vi "Format Pin Name In Error Message.vi"(0 "Pin Name":string[](array[string]), 2 "Parameter Name":string, 5 "Error[]":bool[](array[boolean]), 11 "error in":errorcluster) -> (4 "Error Message":string, 15 "error out":errorcluster)   [LabVIEW 2024, in "devicePowerSequencerCoreLogic.lvlib"]
uses:
  devicePowerSequencerCoreLogic.lvlib
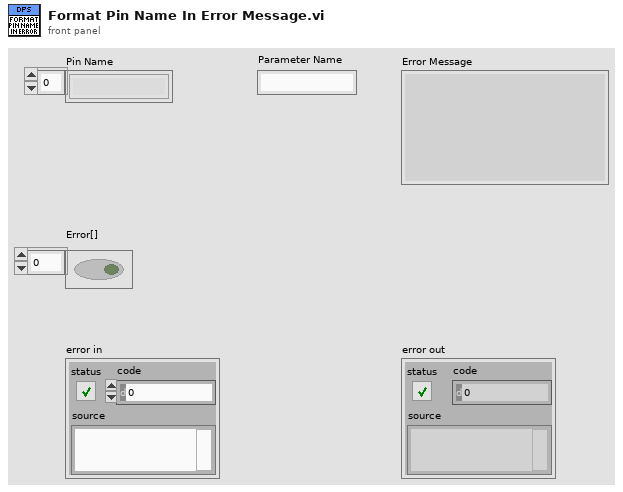
[diagram p1: front panel]
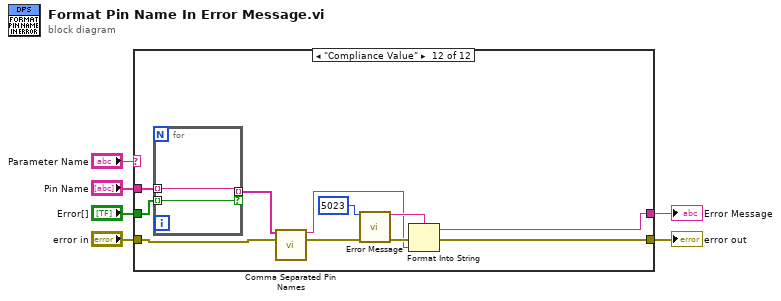
[diagram p0: block diagram]
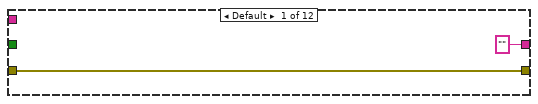
[diagram p2: hidden frame]
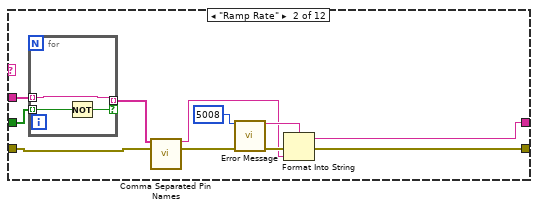
[diagram p3: hidden frame]
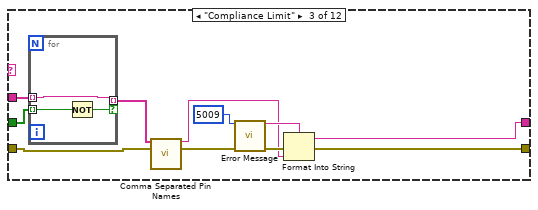
[diagram p4: hidden frame]
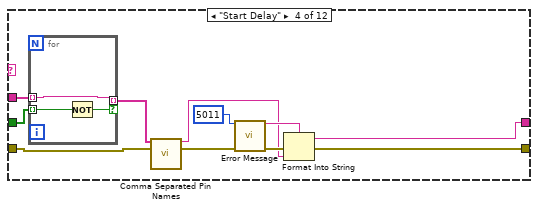
[diagram p5: hidden frame]
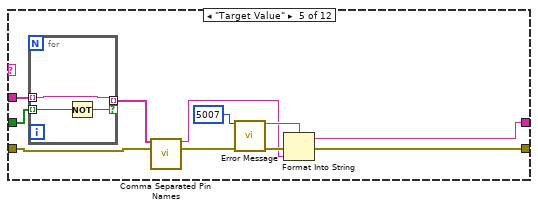
[diagram p6: hidden frame]
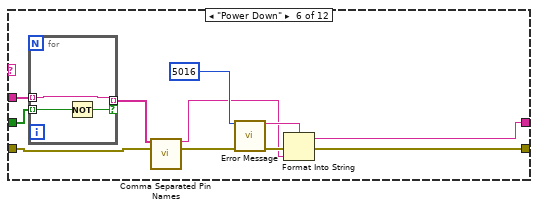
[diagram p7: hidden frame]
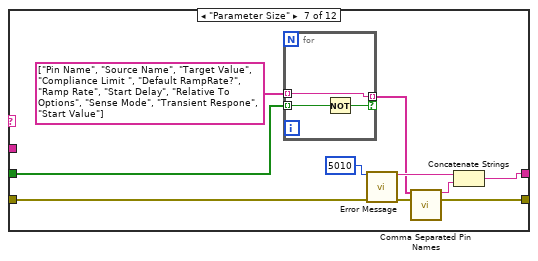
[diagram p8: hidden frame]
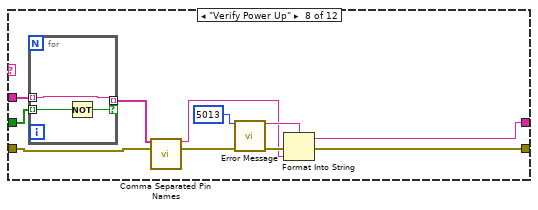
[diagram p9: hidden frame]
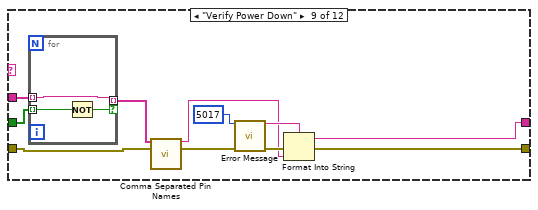
[diagram p10: hidden frame]
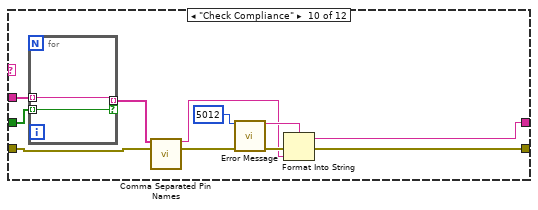
[diagram p11: hidden frame]
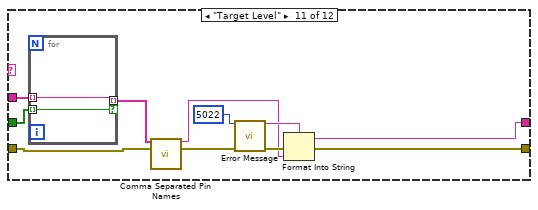
[diagram p12: hidden frame]
diagram:
  n1 = case shown="\"Compliance Value\"" "Parameter Name" {
    tunnel: "Pin Name" -> [_ w19 w33 w47 w61 w75 _ w102 w116 w130 w143 w156]
    tunnel: "Error[]" -> [_ w18 w32 w46 w60 w74 w86 w101 w115 w129 w142 w155]
    tunnel: ["" w17 w31 w45 w59 w73 w87 w100 w114 w128 w141 w154] -> w3
    tunnel: [w7 w16 w30 w44 w58 w72 w80 w99 w113 w127 w140 w153] -> w2
    tunnel: "error in" -> [w7 w9 w23 w37 w51 w65 w83 w92 w108 w120 w133 w146]
    frame Default {
    }
    frame "Ramp Rate" {
      n2 = for {
        tunnel: w19 -> [w22] mode=indexing
        tunnel: w18 -> [w21] mode=indexing
        tunnel: [w22] -> w12 mode=indexing if=w20
        n3 = Not(x=w21) -> (.not. x?=w20:bool)
      }
      n4 = call "Comma Separated Pin Names.vi"("Pin Names"=w12, "error in (no error)"=w9) -> ("PinNames OUT"=w11:string, "error out"=w10:errorcluster)  [unwired: 12 in]
      n5 = call "Error Message.vi"("Error Code"=5008, "error in (no error)"=w10) -> ("Error Message"=w13:string, "error out"=w14:errorcluster)  [unwired: 11 in, 1 out]
      n6 = Format Into String(format string=w13, error in=w14, w11) -> (resulting string=w17:string, error out=w16:errorcluster)  [unwired: 1 in]
    }
    frame "Compliance Limit" {
      n7 = for {
        tunnel: w33 -> [w36] mode=indexing
        tunnel: w32 -> [w35] mode=indexing
        tunnel: [w36] -> w26 mode=indexing if=w34
        n8 = Not(x=w35) -> (.not. x?=w34:bool)
      }
      n9 = call "Comma Separated Pin Names.vi"("Pin Names"=w26, "error in (no error)"=w23) -> ("PinNames OUT"=w25:string, "error out"=w24:errorcluster)  [unwired: 12 in]
      n10 = call "Error Message.vi"("Error Code"=5009, "error in (no error)"=w24) -> ("Error Message"=w28:string, "error out"=w29:errorcluster)  [unwired: 11 in, 1 out]
      n11 = Format Into String(format string=w28, error in=w29, w25) -> (resulting string=w31:string, error out=w30:errorcluster)  [unwired: 1 in]
    }
    frame "Start Delay" {
      n12 = for {
        tunnel: w47 -> [w50] mode=indexing
        tunnel: w46 -> [w49] mode=indexing
        tunnel: [w50] -> w40 mode=indexing if=w48
        n13 = Not(x=w49) -> (.not. x?=w48:bool)
      }
      n14 = call "Comma Separated Pin Names.vi"("Pin Names"=w40, "error in (no error)"=w37) -> ("PinNames OUT"=w39:string, "error out"=w38:errorcluster)  [unwired: 12 in]
      n15 = call "Error Message.vi"("Error Code"=5011, "error in (no error)"=w38) -> ("Error Message"=w41:string, "error out"=w42:errorcluster)  [unwired: 11 in, 1 out]
      n16 = Format Into String(format string=w41, error in=w42, w39) -> (resulting string=w45:string, error out=w44:errorcluster)  [unwired: 1 in]
    }
    frame "Target Value" {
      n17 = for {
        tunnel: w61 -> [w64] mode=indexing
        tunnel: w60 -> [w63] mode=indexing
        tunnel: [w64] -> w54 mode=indexing if=w62
        n18 = Not(x=w63) -> (.not. x?=w62:bool)
      }
      n19 = call "Comma Separated Pin Names.vi"("Pin Names"=w54, "error in (no error)"=w51) -> ("PinNames OUT"=w53:string, "error out"=w52:errorcluster)  [unwired: 12 in]
      n20 = call "Error Message.vi"("Error Code"=5007, "error in (no error)"=w52) -> ("Error Message"=w56:string, "error out"=w57:errorcluster)  [unwired: 11 in, 1 out]
      n21 = Format Into String(format string=w56, error in=w57, w53) -> (resulting string=w59:string, error out=w58:errorcluster)  [unwired: 1 in]
    }
    frame "Power Down" {
      n22 = for {
        tunnel: w75 -> [w78] mode=indexing
        tunnel: w74 -> [w77] mode=indexing
        tunnel: [w78] -> w68 mode=indexing if=w76
        n23 = Not(x=w77) -> (.not. x?=w76:bool)
      }
      n24 = call "Comma Separated Pin Names.vi"("Pin Names"=w68, "error in (no error)"=w65) -> ("PinNames OUT"=w67:string, "error out"=w66:errorcluster)  [unwired: 12 in]
      n25 = call "Error Message.vi"("Error Code"=5016, "error in (no error)"=w66) -> ("Error Message"=w70:string, "error out"=w71:errorcluster)  [unwired: 11 in, 1 out]
      n26 = Format Into String(format string=w70, error in=w71, w67) -> (resulting string=w73:string, error out=w72:errorcluster)  [unwired: 1 in]
    }
    frame "Parameter Size" {
      n27 = for {
        tunnel: w86 -> [w90] mode=indexing
        tunnel: string[] ["Pin Name", "Source Name", "Target Value", "Compliance Limit ", "Default RampRate?", "Ramp Rate", "Start Delay", "Relative To Options", "Sense Mode", "Transient Respone", "Start Value"] -> [w91] mode=indexing
        tunnel: [w91] -> w82 mode=indexing if=w89
        n28 = Not(x=w90) -> (.not. x?=w89:bool)
      }
      n29 = call "Error Message.vi"("Error Code"=5010, "error in (no error)"=w83) -> ("Error Message"=w84:string, "error out"=w79:errorcluster)  [unwired: 11 in, 1 out]
      n30 = call "Comma Separated Pin Names.vi"("Pin Names"=w82, "error in (no error)"=w79) -> ("PinNames OUT"=w81:string, "error out"=w80:errorcluster)  [unwired: 12 in]
      n31 = Concatenate Strings(w84, w81) -> (w87:string)
    }
    frame "Verify Power Up" {
      n32 = for {
        tunnel: w102 -> [w105] mode=indexing
        tunnel: w101 -> [w104] mode=indexing
        tunnel: [w105] -> w95 mode=indexing if=w103
        n33 = Not(x=w104) -> (.not. x?=w103:bool)
      }
      n34 = call "Comma Separated Pin Names.vi"("Pin Names"=w95, "error in (no error)"=w92) -> ("PinNames OUT"=w94:string, "error out"=w93:errorcluster)  [unwired: 12 in]
      n35 = call "Error Message.vi"("Error Code"=5013, "error in (no error)"=w93) -> ("Error Message"=w97:string, "error out"=w96:errorcluster)  [unwired: 11 in, 1 out]
      n36 = Format Into String(format string=w97, error in=w96, w94) -> (resulting string=w100:string, error out=w99:errorcluster)  [unwired: 1 in]
    }
    frame "Verify Power Down" {
      n37 = for {
        tunnel: w116 -> [w119] mode=indexing
        tunnel: w115 -> [w118] mode=indexing
        tunnel: [w119] -> w109 mode=indexing if=w117
        n38 = Not(x=w118) -> (.not. x?=w117:bool)
      }
      n39 = call "Comma Separated Pin Names.vi"("Pin Names"=w109, "error in (no error)"=w108) -> ("PinNames OUT"=w107:string, "error out"=w106:errorcluster)  [unwired: 12 in]
      n40 = call "Error Message.vi"("Error Code"=5017, "error in (no error)"=w106) -> ("Error Message"=w112:string, "error out"=w111:errorcluster)  [unwired: 11 in, 1 out]
      n41 = Format Into String(format string=w112, error in=w111, w107) -> (resulting string=w114:string, error out=w113:errorcluster)  [unwired: 1 in]
    }
    frame "Check Compliance" {
      n42 = for {
        tunnel: w130 -> [w132] mode=indexing
        tunnel: w129 -> [w131] mode=indexing
        tunnel: [w132] -> w123 mode=indexing if=w131
      }
      n43 = call "Comma Separated Pin Names.vi"("Pin Names"=w123, "error in (no error)"=w120) -> ("PinNames OUT"=w122:string, "error out"=w121:errorcluster)  [unwired: 12 in]
      n44 = call "Error Message.vi"("Error Code"=5012, "error in (no error)"=w121) -> ("Error Message"=w126:string, "error out"=w125:errorcluster)  [unwired: 11 in, 1 out]
      n45 = Format Into String(format string=w126, error in=w125, w122) -> (resulting string=w128:string, error out=w127:errorcluster)  [unwired: 1 in]
    }
    frame "Target Level" {
      n46 = for {
        tunnel: w143 -> [w145] mode=indexing
        tunnel: w142 -> [w144] mode=indexing
        tunnel: [w145] -> w136 mode=indexing if=w144
      }
      n47 = call "Comma Separated Pin Names.vi"("Pin Names"=w136, "error in (no error)"=w133) -> ("PinNames OUT"=w135:string, "error out"=w134:errorcluster)  [unwired: 12 in]
      n48 = call "Error Message.vi"("Error Code"=5022, "error in (no error)"=w134) -> ("Error Message"=w139:string, "error out"=w138:errorcluster)  [unwired: 11 in, 1 out]
      n49 = Format Into String(format string=w139, error in=w138, w135) -> (resulting string=w141:string, error out=w140:errorcluster)  [unwired: 1 in]
    }
    frame "Compliance Value" {
      n50 = for {
        tunnel: w156 -> [w158] mode=indexing
        tunnel: w155 -> [w157] mode=indexing
        tunnel: [w158] -> w149 mode=indexing if=w157
      }
      n51 = call "Comma Separated Pin Names.vi"("Pin Names"=w149, "error in (no error)"=w146) -> ("PinNames OUT"=w148:string, "error out"=w147:errorcluster)  [unwired: 12 in]
      n52 = call "Error Message.vi"("Error Code"=5023, "error in (no error)"=w147) -> ("Error Message"=w152:string, "error out"=w151:errorcluster)  [unwired: 11 in, 1 out]
      n53 = Format Into String(format string=w152, error in=w151, w148) -> (resulting string=w154:string, error out=w153:errorcluster)  [unwired: 1 in]
    }
  }
  "Error Message" <- w3
  "error out" <- w2
